vi "G2CPU Rake Lines.vi"(6 "Auto Release (Enabled)":T3={"Auto Release Px 1 (Enabled)"=TRUE, "Auto Release Py 1 (Enabled)"=TRUE, "Auto Release Px 2 (Enabled)"=TRUE, "Auto Release Py 2 (Enabled)"=TRUE, "Auto Release Px 3 (Enabled)"=TRUE, "Auto Release Py 3 (Enabled)"=TRUE, "Auto Release Amount of Lines (Enabled)"=TRUE}, 8 "error in (no error)":errorcluster, 11 "Rake Parameters":T1) -> (0 "error out":errorcluster, 3 "Lines":T2)   [LabVIEW 2024, in "G2CPU Line Profile.lvlib"]
doc: "Create a set of points representing a set of rakes for image processing.\nThe width of the rake is defined by the Point 1 to Point 2 parameters.\nThe length of the rake is defined by the Point 1 to Point 2 parameters.\n\nPoints 1 on the output define the starting point of the lines and Points 2 define the stopping point of the lines.\nThe keys put out define the grouping of the lines to each rake."
uses:
  G2CPU Line Profile.lvlib
  <vilib>/Natan Biesmans/G2CPU GPU and CPU HPC Toolkit/G2CPU Libraries/Arrays/1DArray/u32/1D Array u32.lvclass
  da00906a-c606-4c9d-b3ab-5fe3913f5c92.vi
  5102891f-fe1b-4a86-92fd-1fc4f8e421d2.vi
  206e0866-6077-4d66-9331-fd05babc3295.vi
  c4294105-9b10-401a-880d-43090311ea98.vi
  edcb799f-5326-466a-9748-81893007730a.vi
  6fe21552-c08b-4cc6-9e47-eec4454b2c27.vi
  c98707c9-344b-4084-8106-3c5d35b7e7af.vi
  a71a51f2-f1ac-4743-88d3-77d190704f14.vi
  f90bb481-9117-4697-95de-c99e598d36a8.vi
  843c4b26-1725-4ea9-995a-a7f3be456a06.vi
  8f1c249d-60e2-4233-a983-5733fb4c28e8.vi
  a08def0a-358c-469c-bfdc-17a408e02bf4.vi
  dd15c6ab-5bff-4ac6-babb-c866b3d74303.vi
  2e5a495c-9f7b-42b5-a818-f6f700be2791.vi
  bfc18300-09c0-472a-8fbd-0ede8509d07b.vi
  <vilib>/Natan Biesmans/G2CPU GPU and CPU HPC Toolkit/G2CPU Libraries/Arrays/1DArray/f32/1D Array f32.lvclass
  1cc8f18f-e92e-466b-a53e-c3ffcafd6db7.vi
  2e05728a-c73c-4486-ac1e-57e17aef81c3.vi
  3a05a93a-8157-413f-ac1a-af608df0fd60.vi
  5c735bd4-8f6b-47a4-b0b8-8abdc091b224.vi
  656b9592-5212-4e70-b003-0855a0d8194e.vi
  6e27f1a3-c5cf-432c-9e27-1f4125722014.vi
  <vilib>/Natan Biesmans/G2CPU GPU and CPU HPC Toolkit/G2CPU Libraries/Arrays/Array/Array Prototype.lvclass
  <vilib>/Natan Biesmans/G2CPU GPU and CPU HPC Toolkit/G2CPU Libraries/Arrays/1DArray/s32/1D Array s32.lvclass
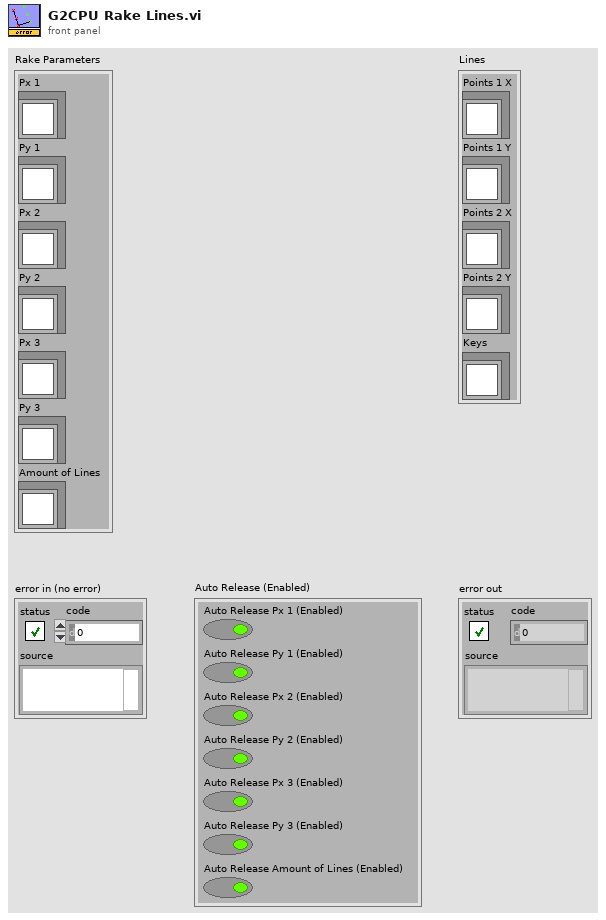
[diagram p1: front panel]
types:
  T1 = cluster{"Px 1":refnum<class "1D Array f32.lvclass">, "Py 1":refnum<class "1D Array f32.lvclass">, "Px 2":refnum<class "1D Array f32.lvclass">, "Py 2":refnum<class "1D Array f32.lvclass">, "Px 3":refnum<class "1D Array f32.lvclass">, "Py 3":refnum<class "1D Array f32.lvclass">, "Amount of Lines":refnum<class "1D Array s32.lvclass">}
  T2 = cluster{"Points 1 X":refnum<class "1D Array f32.lvclass">, "Points 1 Y":refnum<class "1D Array f32.lvclass">, "Points 2 X":refnum<class "1D Array f32.lvclass">, "Points 2 Y":refnum<class "1D Array f32.lvclass">, "Keys":refnum<class "1D Array u32.lvclass">}
  T3 = cluster{"Auto Release Px 1 (Enabled)":bool, "Auto Release Py 1 (Enabled)":bool, "Auto Release Px 2 (Enabled)":bool, "Auto Release Py 2 (Enabled)":bool, "Auto Release Px 3 (Enabled)":bool, "Auto Release Py 3 (Enabled)":bool, "Auto Release Amount of Lines (Enabled)":bool}
  T4 = cluster{"Px 1":refnum<class "1D Array f32.lvclass">, "Py 1":refnum<class "1D Array f32.lvclass">, "Px 2":refnum<class "1D Array f32.lvclass">, "Py 2":refnum<class "1D Array f32.lvclass">, "Keys":refnum<class "1D Array u32.lvclass">}
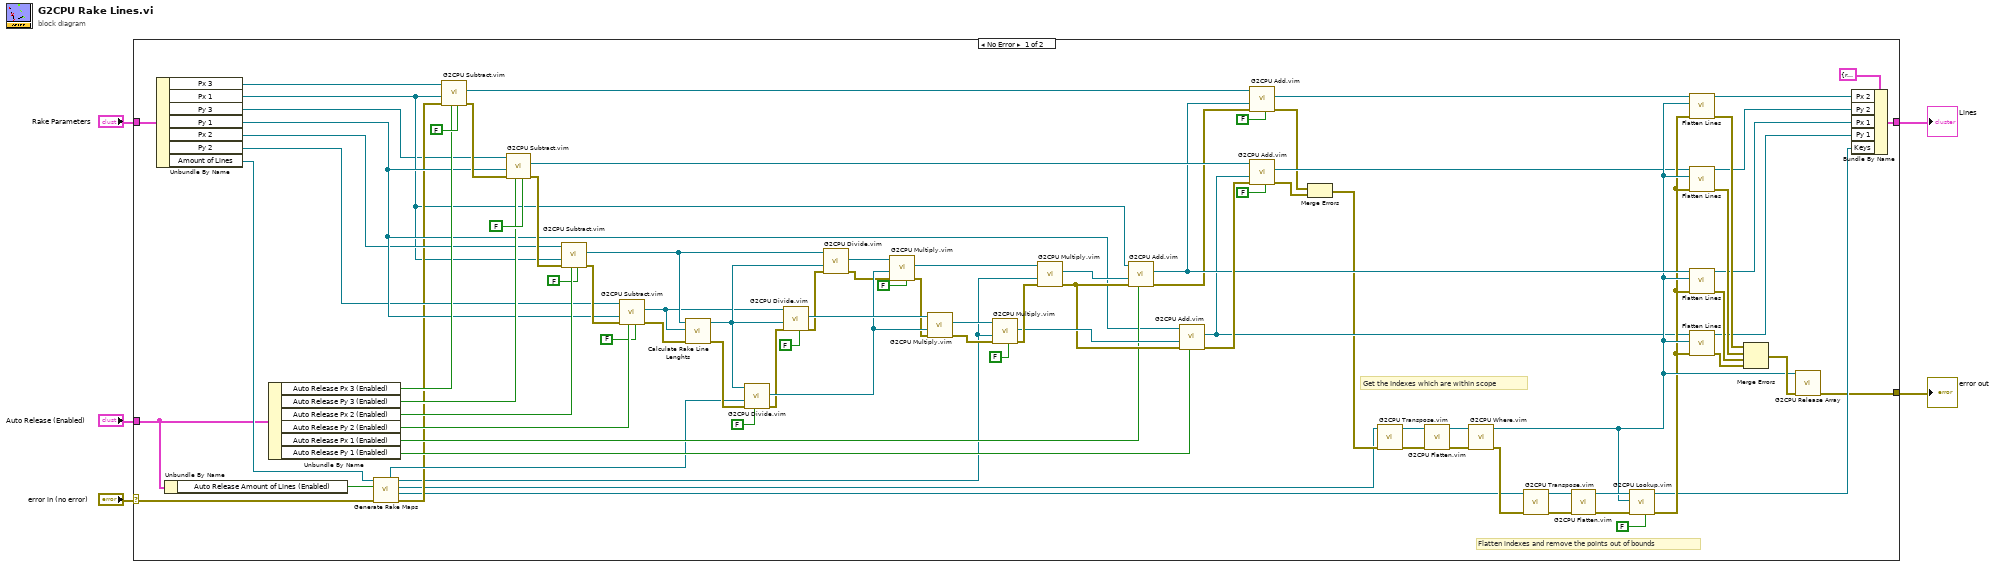
[diagram p0: block diagram]
diagram:
  n1 = case shown="No Error" "error in (no error)" {
    selector: "error in (no error)" -> [w14 w96]
    tunnel: "Auto Release (Enabled)" -> [w13 _]
    tunnel: [w29 _] -> w4
    tunnel: [w27 w96] -> w3
    tunnel: "Rake Parameters" -> [w20 _]
    frame No Error {
      # "Flatten indexes and remove the points out of bounds"
      # "Get the Indexes which are within scope"
      n2 = Unbundle By Name(w20) -> ("Px 3"=w19:refnum<class "1D Array f32.lvclass">, "Px 1"=w7:refnum<class "1D Array f32.lvclass">, "Py 3"=w6:refnum<class "1D Array f32.lvclass">, "Py 1"=w18:refnum<class "1D Array f32.lvclass">, "Px 2"=w17:refnum<class "1D Array f32.lvclass">, "Py 2"=w16:refnum<class "1D Array f32.lvclass">, "Amount of Lines"=w15:refnum<class "1D Array s32.lvclass">)
      n3 = Unbundle By Name(w13) -> ("Auto Release Amount of Lines (Enabled)"=w12:bool)
      n4 = Unbundle By Name(w13) -> ("Auto Release Px 3 (Enabled)"=w72:bool, "Auto Release Py 3 (Enabled)"=w71:bool, "Auto Release Px 2 (Enabled)"=w70:bool, "Auto Release Py 2 (Enabled)"=w69:bool, "Auto Release Px 1 (Enabled)"=w58:bool, "Auto Release Py 1 (Enabled)"=w59:bool)
      n5 = call "Generate Rake Maps.vi"("error in (no error)"=w14, "Auto Release Amount of Lines in Rake (Enabled)"=w12, "Amount of Lines in Rake"=w15) -> ("error out"=w11:errorcluster, "Rake Keys"=w8:refnum<class "2D Array u32.lvclass">, "In Bounds Mask"=w9:refnum<class "2D Array binary.lvclass">, "Line Indexes"=w10:refnum<class "2D Array f32.lvclass">, "Line Divisions"=w57:refnum<class "1D Array f32.lvclass">)  [unwired: 4 in]
      n6 = call "G2CPU Subtract.vim"("Auto Release rhs (Enabled)"=FALSE, "Auto Release lhs (Enabled)"=w72, "error in (no error)"=w11, "Array rhs"=w7, "Array lhs"=w19) -> ("error out"=w77:errorcluster, "Array Result"=w89:refnum<class "1D Array f32.lvclass">)  [unwired: 5 in]
      n7 = call "G2CPU Subtract.vim"("Auto Release rhs (Enabled)"=FALSE, "Auto Release lhs (Enabled)"=w71, "error in (no error)"=w77, "Array rhs"=w18, "Array lhs"=w6) -> ("error out"=w76:errorcluster, "Array Result"=w88:refnum<class "1D Array f32.lvclass">)  [unwired: 5 in]
      n8 = call "G2CPU Subtract.vim"("Auto Release rhs (Enabled)"=FALSE, "Auto Release lhs (Enabled)"=w70, "error in (no error)"=w76, "Array rhs"=w7, "Array lhs"=w17) -> ("error out"=w75:errorcluster, "Array Result"=w22:refnum<class "1D Array f32.lvclass">)  [unwired: 5 in]
      n9 = call "G2CPU Subtract.vim"("Auto Release rhs (Enabled)"=FALSE, "Auto Release lhs (Enabled)"=w69, "error in (no error)"=w75, "Array rhs"=w18, "Array lhs"=w16) -> ("error out"=w23:errorcluster, "Array Result"=w21:refnum<class "1D Array f32.lvclass">)  [unwired: 5 in]
      n10 = call "Calculate Rake Line Lenghts.vi"("error in (no error)"=w23, "Lines Y Distances (non released)"=w21, "Lines X Distances (non released)"=w22) -> ("error out"=w78:errorcluster, "Rake Line Lengths"=w93:refnum<class "1D Array f32.lvclass">)  [unwired: 7 in]
      n11 = call "G2CPU Divide.vim"("Auto Release lhs (Enabled)"=FALSE, "error in (no error)"=w78, "Array rhs"=w57, "Array lhs"=w93) -> ("error out"=w84:errorcluster, "Array Result"=w92:refnum<class "1D Array f32.lvclass">)  [unwired: 6 in]
      n12 = call "G2CPU Divide.vim"("Auto Release rhs (Enabled)"=FALSE, "error in (no error)"=w84, "Array rhs"=w93, "Array lhs"=w21) -> ("error out"=w83:errorcluster, "Array Result"=w94:refnum<class "1D Array f32.lvclass">)  [unwired: 6 in]
      n13 = call "G2CPU Divide.vim"("error in (no error)"=w83, "Array rhs"=w93, "Array lhs"=w22) -> ("error out"=w82:errorcluster, "Array Result"=w95:refnum<class "1D Array f32.lvclass">)  [unwired: 7 in]
      n14 = call "G2CPU Multiply.vim"("Auto Release rhs"=FALSE, "error in (no error)"=w82, "Array rhs"=w92, "Array lhs"=w95) -> ("error out"=w86:errorcluster, "Array Result"=w91:refnum<class "1D Array f32.lvclass">)  [unwired: 6 in]
      n15 = call "G2CPU Multiply.vim"("error in (no error)"=w86, "Array rhs"=w92, "Array lhs"=w94) -> ("error out"=w85:errorcluster, "Array Result"=w90:refnum<class "1D Array f32.lvclass">)  [unwired: 7 in]
      n16 = call "G2CPU Multiply.vim"("Auto Release rhs"=FALSE, "error in (no error)"=w85, "Array rhs"=w10, "Array lhs"=w90) -> ("error out"=w87:errorcluster, "Array Result"=w67:refnum<class "2D Array f32.lvclass">)  [unwired: 6 in]
      n17 = call "G2CPU Multiply.vim"("error in (no error)"=w87, "Array rhs"=w10, "Array lhs"=w91) -> ("error out"=w64:errorcluster, "Array Result"=w65:refnum<class "2D Array f32.lvclass">)  [unwired: 7 in]
      n18 = call "G2CPU Add.vim"("Auto Release lhs (Enabled)"=w58, "error in (no error)"=w64, "Array rhs"=w65, "Array lhs"=w7) -> ("error out"=w62:errorcluster, "Array Result"=w63:refnum<class "2D Array f32.lvclass">)  [unwired: 6 in]
      n19 = call "G2CPU Add.vim"("Auto Release lhs (Enabled)"=w59, "error in (no error)"=w64, "Array rhs"=w67, "Array lhs"=w18) -> ("error out"=w66:errorcluster, "Array Result"=w34:refnum<class "2D Array f32.lvclass">)  [unwired: 6 in]
      n20 = call "G2CPU Add.vim"("Auto Release rhs (Enabled)"=FALSE, "error in (no error)"=w62, "Array rhs"=w63, "Array lhs"=w89) -> ("error out"=w25:errorcluster, "Array Result"=w31:refnum<class "2D Array f32.lvclass">)  [unwired: 6 in]
      n21 = call "G2CPU Add.vim"("Auto Release rhs (Enabled)"=FALSE, "error in (no error)"=w66, "Array rhs"=w34, "Array lhs"=w88) -> ("error out"=w26:errorcluster, "Array Result"=w30:refnum<class "2D Array f32.lvclass">)  [unwired: 6 in]
      n22 = Merge Errors(w25, w26) -> (w24:errorcluster)
      n23 = call "G2CPU Transpose.vim"("error in (no error)"=w24, "Array In"=w9) -> ("error out"=w45:errorcluster, "Array out"=w55:refnum<class "2D Array binary.lvclass">)  [unwired: 8 in]
      n24 = call "G2CPU Flatten.vim"("error in (no error)"=w45, "Array In"=w55) -> ("error out"=w44:errorcluster, "Array out"=w54:refnum<class "1D Array binary.lvclass">)  [unwired: 8 in]
      n25 = call "G2CPU Where.vim"("error in (no error)"=w44, "Array in"=w54) -> ("error out"=w41:errorcluster, "Non Zero Indices"=w46:refnum<class "1D Array u32.lvclass">)  [unwired: 8 in]
      n26 = call "G2CPU Transpose.vim"("error in (no error)"=w41, "Array In"=w8) -> ("error out"=w43:errorcluster, "Array out"=w56:refnum<class "2D Array u32.lvclass">)  [unwired: 8 in]
      n27 = call "G2CPU Flatten.vim"("error in (no error)"=w43, "Array In"=w56) -> ("error out"=w42:errorcluster, "Array out"=w52:refnum<class "1D Array u32.lvclass">)  [unwired: 8 in]
      n28 = call "G2CPU Lookup.vim"("Auto Release Indices (Enabled)"=FALSE, "error in (no error)"=w42, "Indices (1D)"=w46, "Array In"=w52) -> ("error out"=w40:errorcluster, "Indexed Array"=w28:refnum<class "1D Array u32.lvclass">)  [unwired: 6 in]
      n29 = call "Flatten Lines.vi"("error in (no error)"=w40, "Valid Point Indexes (flattened)"=w46, "Lines In"=w31) -> ("error out"=w51:errorcluster, "Flattened Lines Out"=w38:refnum<class "1D Array f32.lvclass">)  [unwired: 7 in]
      n30 = call "Flatten Lines.vi"("error in (no error)"=w40, "Valid Point Indexes (flattened)"=w46, "Lines In"=w30) -> ("error out"=w50:errorcluster, "Flattened Lines Out"=w37:refnum<class "1D Array f32.lvclass">)  [unwired: 7 in]
      n31 = call "Flatten Lines.vi"("error in (no error)"=w40, "Valid Point Indexes (flattened)"=w46, "Lines In"=w63) -> ("error out"=w49:errorcluster, "Flattened Lines Out"=w36:refnum<class "1D Array f32.lvclass">)  [unwired: 7 in]
      n32 = call "Flatten Lines.vi"("error in (no error)"=w40, "Valid Point Indexes (flattened)"=w46, "Lines In"=w34) -> ("error out"=w48:errorcluster, "Flattened Lines Out"=w35:refnum<class "1D Array f32.lvclass">)  [unwired: 7 in]
      n33 = Merge Errors(w51, w50, w49, w48) -> (w47:errorcluster)
      n34 = call <vilib>:"G2CPU Release Array.vi"("error in (no error)"=w47, "Array in"=w46) -> ("error out"=w27:errorcluster)  [unwired: 9 in]
      n35 = Bundle By Name(cluster=T4 {"Px 1"=refnum, "Py 1"=refnum, "Px 2"=refnum, "Py 2"=refnum, "Keys"=refnum} ("Cluster"), "Px 2"=w38, "Py 2"=w37, "Px 1"=w36, "Py 1"=w35, "Keys"=w28) -> (w29:T4)
    }
    frame Error {
    }
  }
  "Lines" <- w4
  "error out" <- w3
